vi "PXI-Synchronize Tasks.vi"(0 "Task Array":refnum<k21>[](array[refnum]), 11 "error in (no error)":errorcluster) -> (15 "error out":errorcluster)   [LabVIEW 2015]
uses:
  <vilib>/DAQmx/configure/trigger.llb/DAQmx Start Trigger (Digital Edge).vi
  <resource>/objmgr/daqmx.rc
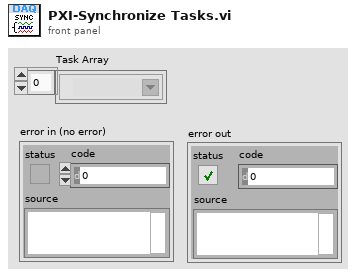
[diagram p1: front panel]
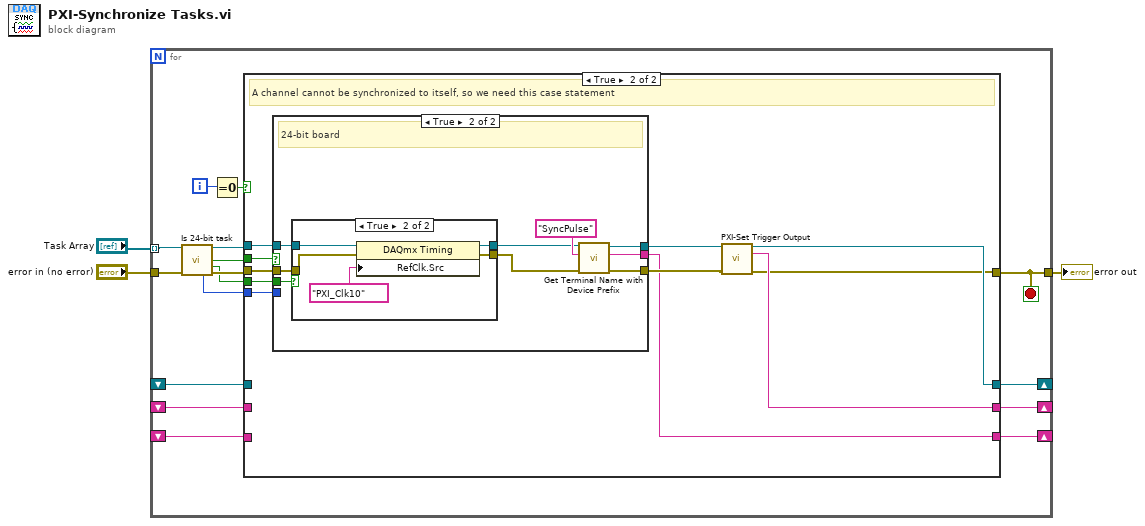
[diagram p0: block diagram]
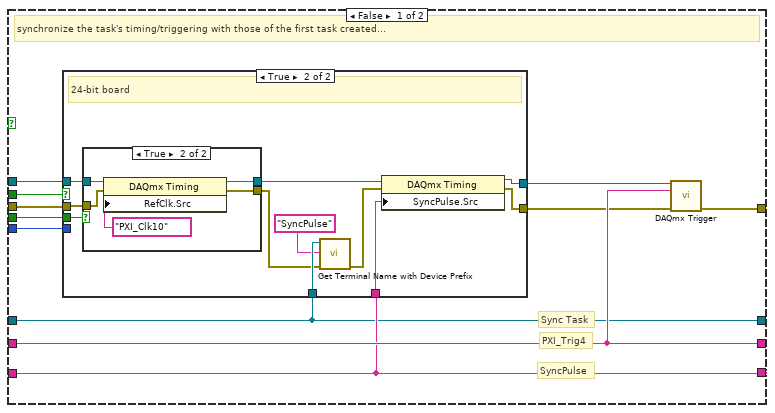
[diagram p2: hidden frame]
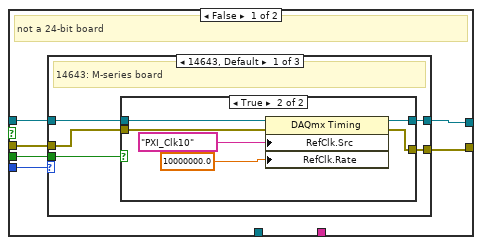
[diagram p3: hidden frame]
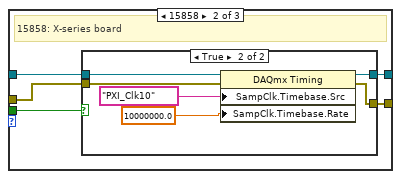
[diagram p5: hidden frame]
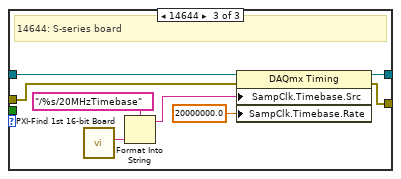
[diagram p7: hidden frame]
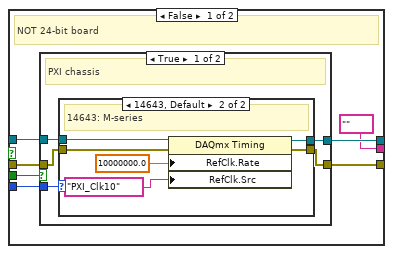
[diagram p9: hidden frame]
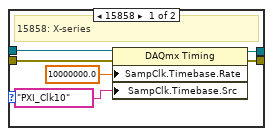
[diagram p10: hidden frame]
diagram:
  n1 = for {
    tunnel: "Task Array" -> [w19] mode=indexing
    shift-right: [w11] -> _
    shift-left: _ -> [w8]
    shift-right: [w10] -> _
    shift-left: _ -> [w7]
    shift-right: [w9] -> _
    shift-left: _ -> [w6]
    tunnel: [w5] -> w3
    tunnel: "error in (no error)" -> [w4]
    i -> [w13]
    stop <- w5 stop-if-true
    n2 = call "Is 24-bit task.vi"("task"=w19, "error in (no error)"=w4) -> ("task out"=w18:refnum<k21>, "is 24bit?"=w17:bool, "PXI?"=w15:bool, "Product Category"=w14:i32, "error out"=w16:errorcluster)  [unwired: 8 in, 1 out]
    n3 = Equal To 0?(x=w13) -> (x = 0?=w12:bool)
    n4 = case shown="True" w12 {
      tunnel: w16 -> [w28 w92]
      tunnel: [w30 w94] -> w5
      tunnel: [w22 w99] -> w11
      tunnel: w8 -> [w22 _]
      tunnel: [w29 w95] -> w10
      tunnel: w7 -> [w29 _]
      tunnel: [w27 w96] -> w9
      tunnel: w6 -> [w27 _]
      tunnel: w18 -> [w23 w93]
      tunnel: w17 -> [w24 w91]
      tunnel: w14 -> [w21 w90]
      tunnel: w15 -> [w20 w89]
      frame False {
        # "SyncPulse"
        # "PXI_Trig4"
        # "Sync Task"
        # "synchronize the task's timing/triggering with those of the first task created..."
        n5 = case shown="True" w24 {
          tunnel: [w34 w81] -> w26
          tunnel: [w35 w80] -> w25
          tunnel: w22 -> [_ w79]
          tunnel: w28 -> [w32 w78]
          tunnel: w27 -> [_ w77]
          tunnel: w23 -> [w33 w72]
          tunnel: w21 -> [w36 _]
          tunnel: w20 -> [w31 w71]
          frame False {
            # "not a 24-bit board"
            n6 = case shown="14643, Default" w36 {
              tunnel: [w41 w54 w70] -> w34
              tunnel: [w40 w53 w69] -> w35
              tunnel: w33 -> [w39 w52 w67]
              tunnel: w32 -> [w38 w51 w66]
              tunnel: w31 -> [w37 w50 _]
              frame 14643, Default {
                # "14643: M-series board"
                n7 = case shown="True" w37 {
                  tunnel: [w43 w49] -> w41
                  tunnel: [w42 w48] -> w40
                  tunnel: w39 -> [w43 w45]
                  tunnel: w38 -> [w42 w44]
                  frame False {
                  }
                  frame True {
                    n8 = property class="DAQmx Timing"(reference=w45, error in=w44, "RefClk.Src"=tag "PXI_Clk10", "RefClk.Rate"=10000000.0) -> (reference out=w49:refnum<k21>, error out=w48:errorcluster)
                  }
                }
              }
              frame 15858 {
                # "15858: X-series board"
                n9 = case shown="True" w50 {
                  tunnel: [w56 w62] -> w54
                  tunnel: [w55 w61] -> w53
                  tunnel: w52 -> [w56 w58]
                  tunnel: w51 -> [w55 w57]
                  frame False {
                  }
                  frame True {
                    n10 = property class="DAQmx Timing"(reference=w58, error in=w57, "SampClk.Timebase.Src"=tag "PXI_Clk10" ("RefClk.Src"), "SampClk.Timebase.Rate"=10000000.0) -> (reference out=w62:refnum<k21>, error out=w61:errorcluster)
                  }
                }
              }
              frame 14644 {
                # "14644: S-series board"
                n11 = call "PXI-Find 1st 16-bit Board.vi"() -> ("DAQmx Device Name"=w63:tag)  [unwired: 9 in, 2 out]
                n12 = Format Into String(format string="/%s/20MHzTimebase", w63) -> (resulting string=w64:string)  [unwired: 2 in, 1 out]
                n13 = property class="DAQmx Timing"(reference=w67, error in=w66, "SampClk.Timebase.Src"=w64, "SampClk.Timebase.Rate"=20000000.0) -> (reference out=w70:refnum<k21>, error out=w69:errorcluster)
              }
            }
          }
          frame True {
            # "24-bit board"
            n14 = case shown="True" w71 {
              tunnel: w78 -> [w82 w88]
              tunnel: [w82 w87] -> w74
              tunnel: [w83 w86] -> w73
              tunnel: w72 -> [w83 w85]
              frame False {
              }
              frame True {
                n15 = property class="DAQmx Timing"(reference=w85, error in=w88, "RefClk.Src"=tag "PXI_Clk10") -> (reference out=w86:refnum<k21>, error out=w87:errorcluster)
              }
            }
            n16 = call "Get Terminal Name with Device Prefix.vi"("error in (no error)"=w74, "Local Terminal Name"="SyncPulse", "task/channels in"=w79) -> ("error out"=w75:errorcluster)  [unwired: 6 in, 2 out]
            n17 = property class="DAQmx Timing"(reference=w73, error in=w75, "SyncPulse.Src"=w77) -> (reference out=w81:refnum<k21>, error out=w80:errorcluster)
          }
        }
        n18 = call-poly <vilib>:"DAQmx Trigger.vi"("task/channels in"=w26, "source"=w29, "error in"=w25) -> ("error out"=w30:errorcluster)  [unwired: 11 in, 1 out]
      }
      frame True {
        # "A channel cannot be synchronized to itself, so we need this case statement"
        n19 = case shown="True" w91 {
          tunnel: [w105 w134] -> w97
          tunnel: w93 -> [w106 w128]
          tunnel: [w104 w133] -> w98
          tunnel: w92 -> [w103 w127]
          tunnel: [tag "" ("Terminal Name with Device Prefix") w132] -> w96
          tunnel: w90 -> [w100 _]
          tunnel: w89 -> [w101 w126]
          frame False {
            # "NOT 24-bit board"
            n20 = case shown="True" w101 {
              tunnel: w106 -> [w111 w125]
              tunnel: [w110 w125] -> w105
              tunnel: [w109 w124] -> w104
              tunnel: w103 -> [w108 w124]
              tunnel: w100 -> [w107 _]
              frame True {
                # "PXI chassis"
                n21 = case shown="14643, Default" w107 {
                  tunnel: w111 -> [w117 w123]
                  tunnel: [w116 w122] -> w110
                  tunnel: [w115 w121] -> w109
                  tunnel: w108 -> [w114 w120]
                  frame 15858 {
                    # "15858: X-series"
                    n22 = property class="DAQmx Timing"(reference=w117, error in=w114, "SampClk.Timebase.Rate"=10000000.0, "SampClk.Timebase.Src"=tag "PXI_Clk10" ("RefClk.Src")) -> (reference out=w116:refnum<k21>, error out=w115:errorcluster)
                  }
                  frame 14643, Default {
                    # "14643: M-series"
                    n23 = property class="DAQmx Timing"(reference=w123, error in=w120, "RefClk.Rate"=10000000.0, "RefClk.Src"=tag "PXI_Clk10") -> (reference out=w122:refnum<k21>, error out=w121:errorcluster)
                  }
                }
              }
              frame False {
                # "NOT PXI chassis"
              }
            }
          }
          frame True {
            # "24-bit board"
            n24 = case shown="True" w126 {
              tunnel: [w136 w141] -> w130
              tunnel: [w135 w140] -> w129
              tunnel: w128 -> [w136 w139]
              tunnel: w127 -> [w135 w138]
              frame False {
              }
              frame True {
                n25 = property class="DAQmx Timing"(reference=w139, error in=w138, "RefClk.Src"=tag "PXI_Clk10") -> (reference out=w141:refnum<k21>, error out=w140:errorcluster)
              }
            }
            n26 = call "Get Terminal Name with Device Prefix.vi"("error in (no error)"=w129, "Local Terminal Name"="SyncPulse", "task/channels in"=w130) -> ("error out"=w133:errorcluster, "Terminal Name with Device Prefix"=w132:tag, "task out"=w134:refnum<k21>)  [unwired: 6 in]
          }
        }
        n27 = call "PXI-Set Trigger Output.vi"("Task in"=w97, "error in (no error)"=w98) -> ("Task out"=w99:refnum<k21>, "Trigger Terminal"=w95:tag, "error out"=w94:errorcluster)  [unwired: 11 in]
      }
    }
  }
  "error out" <- w3
